vi "getVXMfromIndex.vi"(8 "error in (no error)":errorcluster, 9 "Subsystem 1, 2, 3":i32=2, 11 "sub-systems in":refnum<class "sub-systems.lvclass">) -> (0 "error out":errorcluster, 1 "All Axes this subsystem":T1(array[cluster]), 2 "VXMx2 out":refnum<class "VXMx2.lvclass">, 3 "sub-systems out":refnum<class "sub-systems.lvclass">, 5 "Sub-syst number":i32)   [LabVIEW 2018, in "sub-systems.lvclass"]
doc: "return the VXM axis (X, Y, Z, T),\nthe VXM system containing the Axis\nand the sub-syst. number (1-3)"
uses:
  sub-systems.lvclass
  VSMx2/VXMx2.lvclass
  sub-systems.lvclass/sub-systems.ctl
panel:
  # "This .ctl maybe shouldn't be \ncoupled up this high"
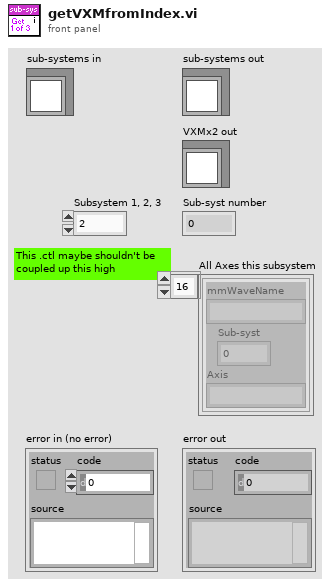
[diagram p1: front panel]
types:
  T1 = cluster{"mmWaveName":string, "Sub-syst":i32, "Axis":string}[]
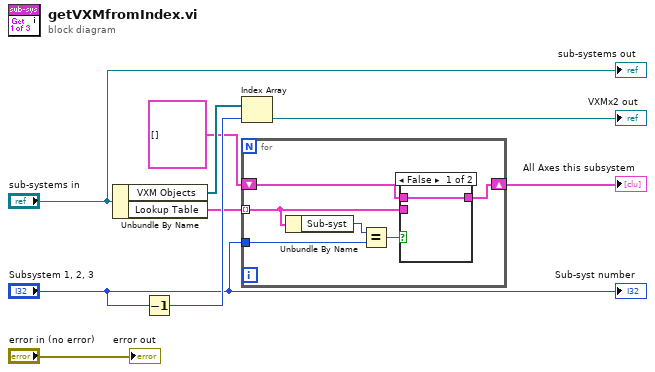
[diagram p0: block diagram]
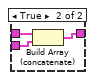
[diagram p2: hidden frame]
diagram:
  n1 = Unbundle By Name("sub-systems in") -> ("VXM Objects"=w7:refnum<class "VXMx2.lvclass">[], "Lookup Table"=w4:T1)
  n2 = Decrement(x="Subsystem 1, 2, 3") -> (x-1=w5:i32)
  n3 = Index Array(array=w7, index=w5) -> (element=→"VXMx2 out":refnum<class "VXMx2.lvclass">)
  n4 = for {
    tunnel: w4 -> [w15] mode=indexing
    shift-right: [w12] -> w2
    shift-left: T1 [] -> [w11]
    tunnel: "Subsystem 1, 2, 3" -> [w13]
    n5 = Unbundle By Name(w15) -> ("Sub-syst"=w14:i32)
    n6 = Equal?(x=w14, y=w13) -> (x = y?=w10:bool)
    n7 = case shown="False" w10 {
      tunnel: w15 -> [_ w19]
      tunnel: [w16 w18] -> w12
      tunnel: w11 -> [w16 w17]
      frame False {
      }
      frame True {
        n8 = Build Array (concatenate)(w17, w19) -> (w18:T1)
      }
    }
  }
  "All Axes this subsystem" <- w2
  "error out" <- "error in (no error)"
  "sub-systems out" <- "sub-systems in"
  "Sub-syst number" <- "Subsystem 1, 2, 3"
